vi "SimpleVariance.vi"(0 "X":dbl[](array[numeric])) -> (2 "variance":dbl[](array[numeric]), 3 "mean":dbl format="%0.2f")   [LabVIEW 2016]
uses:
  <vilib>/Analysis/baseanly.llb/Mean (DBL).vi
  <vilib>/Analysis/NI_AALBase.lvlib
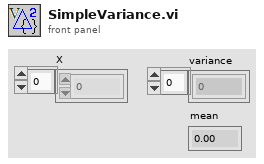
[diagram p1: front panel]
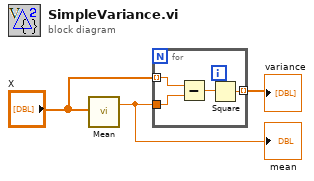
[diagram p0: block diagram]
diagram:
  n1 = call-poly <vilib>:"Mean.vi"("X"="X") -> ("mean"=w3:dbl)  [unwired: 1 out]
  "mean" <- w3
  n2 = for {
    tunnel: "X" -> [w7] mode=indexing
    tunnel: w3 -> [w6]
    tunnel: [w4] -> w2 mode=indexing
    n3 = Subtract(x=w7, y=w6) -> (x-y=w5:dbl)
    n4 = Square(x=w5) -> (x^2=w4:dbl)
  }
  "variance" <- w2
